vi "Get Name (Instance).vi"(8 "error in (no error)":errorcluster, 11 "Command Actor in":refnum<class "Command Actor.lvclass">) -> (0 "error out":errorcluster, 2 "Name (Instance)":string, 3 "Command Actor out":refnum<class "Command Actor.lvclass">)   [LabVIEW 2014, in "Robot Actor Framework.lvlib" / "Command Actor.lvlib" / "Command Actor.lvclass"]
uses:
  Command Actor.lvclass
  Command Actor.lvclass/Command Actor.ctl
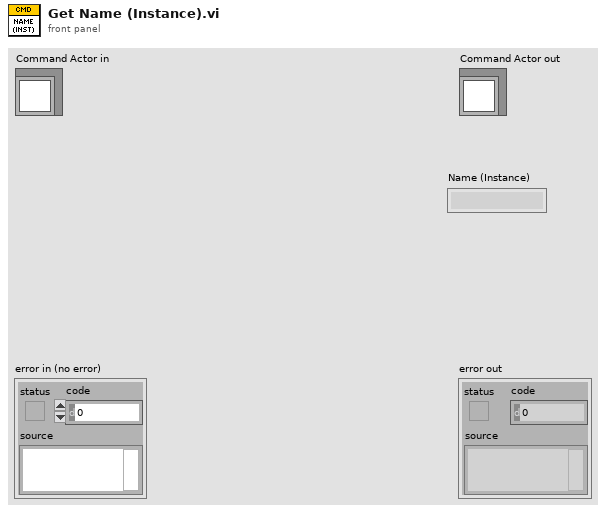
[diagram p1: front panel]
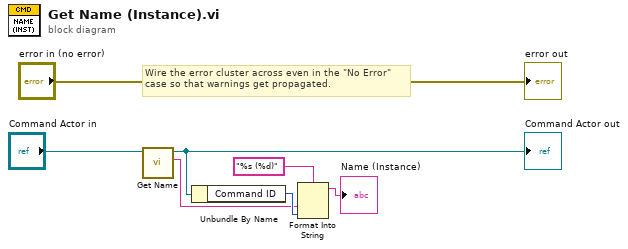
[diagram p0: block diagram]
diagram:
  # "Wire the error cluster across even in the \"No Error\"\ncase so that warnings get propagated."
  n1 = call-dynamic "Get Name.vi"("Command Actor in"="Command Actor in") -> ("Command Name"=w1:string, "Command Actor out"=w5:refnum<class "Command Actor.lvclass">)  [unwired: 8 in, 1 out]
  "Command Actor out" <- w5
  n2 = Unbundle By Name(w5) -> ("Command ID"=w2:u32)
  n3 = Format Into String(format string="%s (%d)", w1, w2) -> (resulting string=→"Name (Instance)":string)  [unwired: 2 in, 1 out]
  "error out" <- "error in (no error)"
